vi "doT2.vi"(10 "parameters_recenter":T5={"input_xyz"={"X_um"=0.0, "Y_um"=0.0, "Z_um"=0.0}, "recenter"=FALSE, "recenter_s"=3}, 11 "T1_parameters":T6) -> (0 "triggers":u32[][](array[numeric]), 1 "std_deviation":dbl[](array[numeric]), 2 "T1 curve":cluster{dbl[], "dark_time_us":dbl[]}(graph), 3 "timetags":u32[][](array[numeric]), 5 "position_xyz":T4, 7 "mini_scan":T3)   [LabVIEW 2018]
uses:
  <vilib>/Analysis/NI_AALBase.lvlib
panel:
  in  "parameters_z-scan":T1={"dwell_time_ms"=2.0, "q_steps"=5, "span_um"=1.0, "refocus"=TRUE}
  in  "parameters_xy-scan":T2={"image_size_xy_um"=2.0, "frame_size_xy_px"=7, "dwell_time_ms"=0.5}
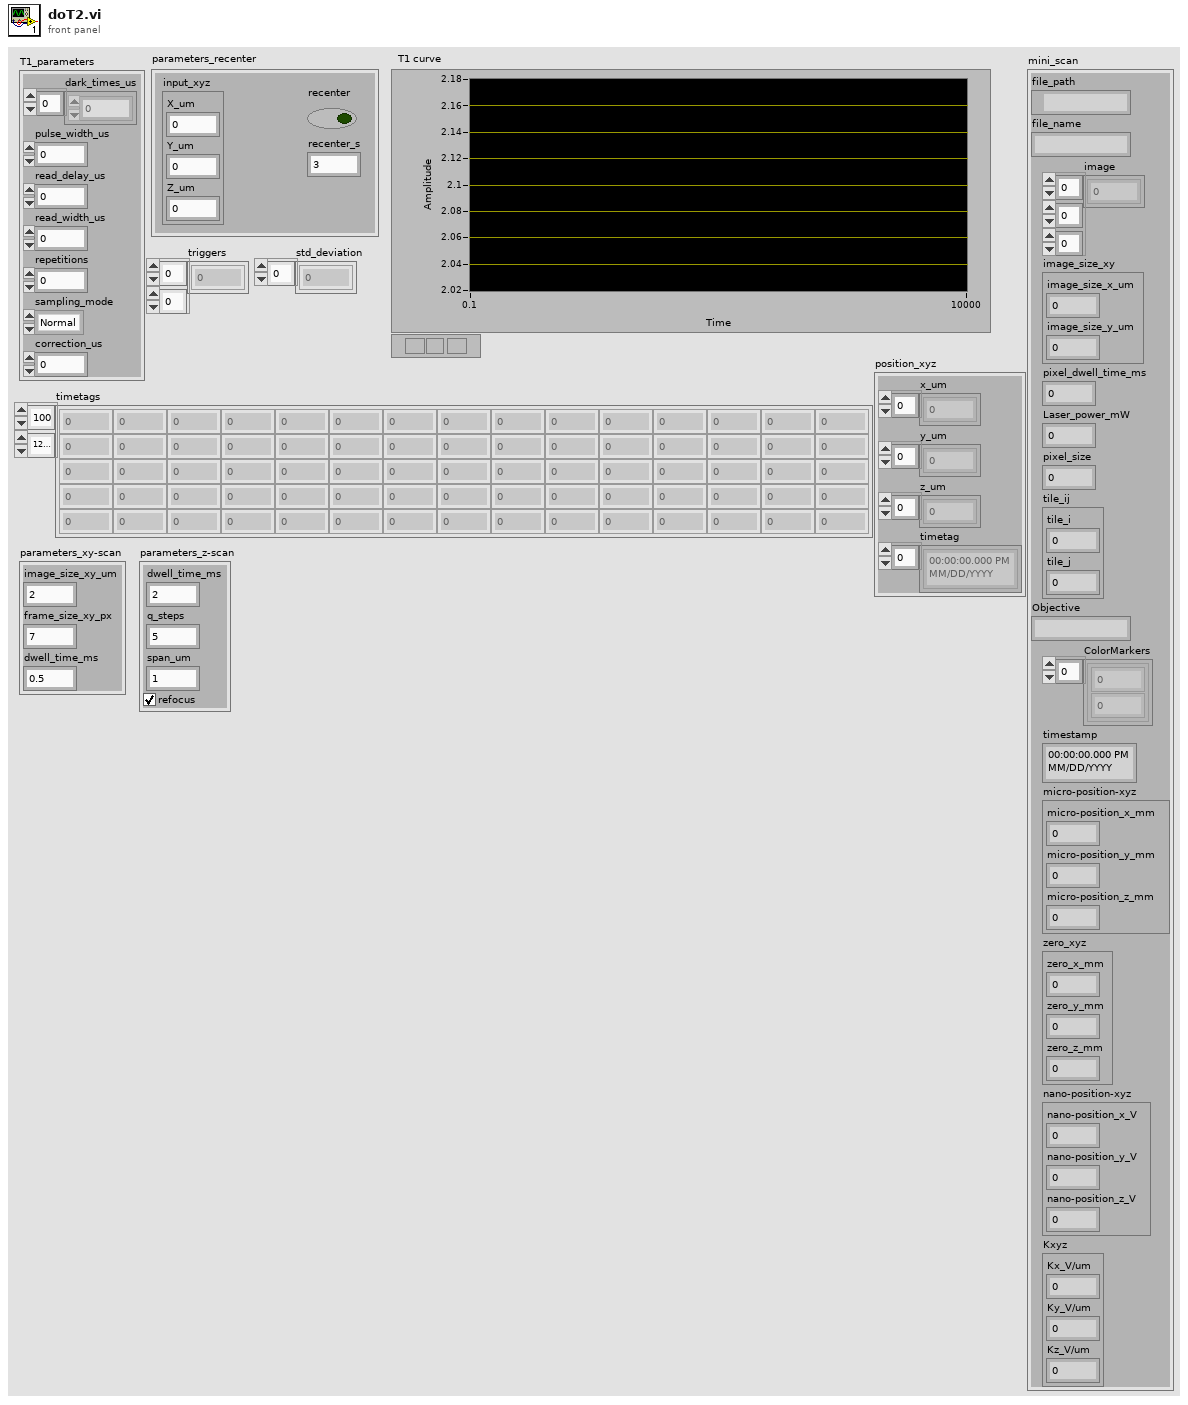
[diagram p1: front panel]
types:
  T1 = cluster{"dwell_time_ms":dbl, "q_steps":u32, "span_um":dbl, "refocus":bool}
  T2 = cluster{"image_size_xy_um":dbl, "frame_size_xy_px":u32, "dwell_time_ms":dbl}
  T3 = cluster{"file_path":path, "file_name":string, "image":dbl[][][], "image_size_xy":cluster{"image_size_x_um":sgl, "image_size_y_um":sgl}, "pixel_dwell_time_ms":sgl, "Laser_power_mW":sgl, "pixel_size":dbl, "tile_ij":cluster{"tile_i":i32, "tile_j":i32}, "Objective":string, "ColorMarkers":cluster{dbl, u32}[], "timestamp":timestamp, "micro-position-xyz":cluster{"micro-position_x_mm":sgl, "micro-position_y_mm":sgl, "micro-position_z_mm":sgl}, "zero_xyz":cluster{"zero_x_mm":dbl, "zero_y_mm":dbl, "zero_z_mm":dbl}, "nano-position-xyz":cluster{"nano-position_x_V":sgl, "nano-position_y_V":sgl, "nano-position_z_V":sgl}, "Kxyz":cluster{"Kx_V/um":sgl, "Ky_V/um":sgl, "Kz_V/um":sgl}}
  T4 = cluster{"x_um":sgl[], "y_um":sgl[], "z_um":sgl[], "timetag":timestamp[]}
  T5 = cluster{"input_xyz":cluster{"X_um":sgl, "Y_um":sgl, "Z_um":sgl}, "recenter":bool, "recenter_s":u32}
  T6 = cluster{"dark_times_us":dbl[], "pulse_width_us":dbl, "read_delay_us":dbl, "read_width_us":dbl, "repetitions":i32, "sampling_mode":enum16{"Normal", "Sweep"}, "correction_us":dbl}
  T7 = cluster{"Instruct Data":i32, "Op Code":i32, "Flags":bool[], "Comments":string, "Time":dbl}[][]
  T8 = cluster{"nano-position_X_um":sgl, "nano-position_Y_um":sgl, "nano-position Z_um":sgl}
  T9 = cluster{"nano-position_X_um":sgl, "nano-position_Y_um":sgl, "nano-position Z_um":sgl}[]
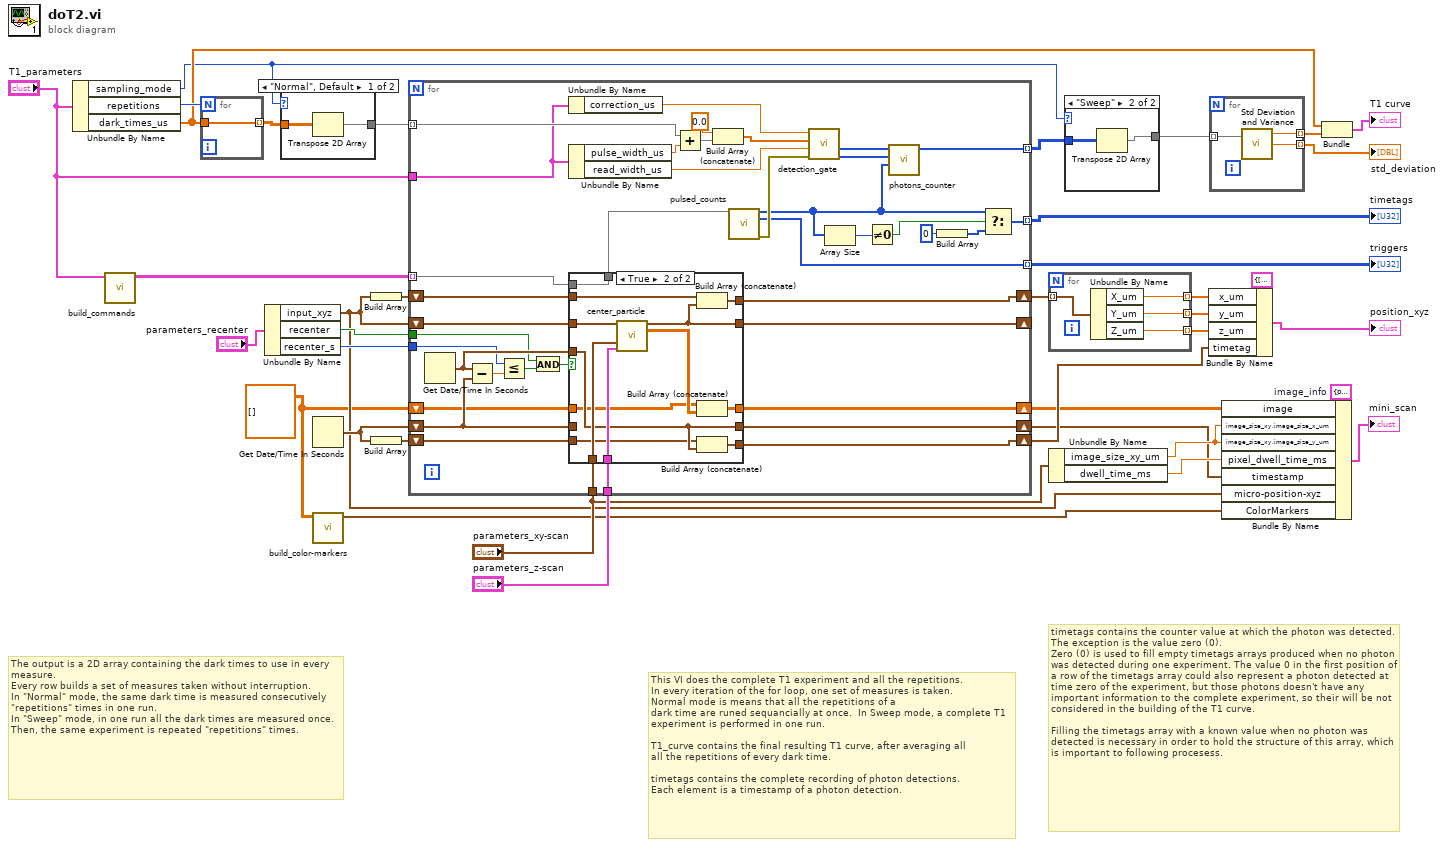
[diagram p0: block diagram]
diagram:
  w2 = dbl[][][] []
  w10 = T3 {"file_path"=path "", "file_name"="", "image"=[], "image_size_xy"={"image_size_x_um"=1.0, "image_size_y_um"=1.0}, "pixel_dwell_time_ms"=1.0, "Laser_power_mW"=1.0, "pixel_size"=0.0, "tile_ij"={"tile_i"=0, "tile_j"=0}, "Objective"="", "ColorMarkers"=[], "timestamp"=timestamp(0 s since 1904-01-01), "micro-position-xyz"={"micro-position_x_mm"=1.0, "micro-position_y_mm"=1.0, "micro-position_z_mm"=1.0}, "zero_xyz"={"zero_x_mm"=0.0, "zero_y_mm"=0.0, "zero_z_mm"=0.0}, "nano-position-xyz"={"nano-position_x_V"=1.0, "nano-position_y_V"=1.0, "nano-position_z_V"=1.0}, "Kxyz"={"Kx_V/um"=1.0, "Ky_V/um"=1.0, "Kz_V/um"=1.0}}  # image_info
  # "timetags contains the counter value at which the photon was detected. The exception is the value zero (0).\nZero (0) is used to fill empty timetags arrays produced when no photon was detected during one experiment. The value 0 in the first position of a row of the timetags array could also represent a photon detected at time zero of the experiment, but those photons doesn't have any important information to the complete experiment, so their will be not considered in the building of the T1 curve.\n\nFilling the timetags array with a known value when no photon was detected is necessary in order to hold the structure of this array, which is important to following procesess."
  # "This VI does the complete T1 experiment and all the repetitions.\nIn every iteration of the for loop, one set of measures is taken.\nNormal mode is means that all the repetitions of a\ndark time are runed sequancially at once.  In Sweep mode, a complete T1 experiment is performed in one run.\n\nT1_curve contains the final resulting T1 curve, after averaging all\nall the repetitions of every dark time.\n\ntimetags contains the complete recording of photon detections.\nEach element is a timestamp of a photon detection."
  # "The output is a 2D array containing the dark times to use in every measure.\nEvery row builds a set of measures taken without interruption.\nIn \"Normal\" mode, the same dark time is measured consecutively \"repetitions\" times in one run.\nIn \"Sweep\" mode, in one run all the dark times are measured once. Then, the same experiment is repeated \"repetitions\" times."
  n1 = Unbundle By Name("T1_parameters") -> ("sampling_mode"=w30:enum16{"Normal", "Sweep"}, "repetitions"=w36:i32, "dark_times_us"=w32:dbl[])
  n2 = call "build_commands.vi"("T1_parameters"="T1_parameters") -> ("instructions_array"=w38:T7)  [unwired: 10 in]
  n3 = for {
    N: w36 -> [_]
    tunnel: w32 -> [w39]
    tunnel: [w39] -> w35 mode=indexing
  }
  n4 = Unbundle By Name("parameters_recenter") -> ("input_xyz"=w3:cluster{"X_um":sgl, "Y_um":sgl, "Z_um":sgl}, "recenter"=w22:bool, "recenter_s"=w23:u32)
  n5 = case shown="\"Normal\", Default" w30 {
    tunnel: w35 -> [w41 w42]
    tunnel: [w40 w42] -> w37
    frame "Normal", Default {
      n6 = Transpose 2D Array(2D array=w41) -> (transposed array=w40:dbl[][])
    }
    frame "Sweep" {
    }
  }
  n7 = Get Date/Time In Seconds() -> (seconds since 1Jan1904=w18:timestamp)
  n8 = call "build_color-markers.vi"("images"=w2) -> ("color_markers"=w1:cluster{dbl, u32}[])  [unwired: 10 in]
  n9 = Build Array(w3) -> (w20:cluster{"X_um":sgl, "Y_um":sgl, "Z_um":sgl}[])
  n10 = Build Array(w18) -> (w19:timestamp[])
  n11 = for {
    tunnel: w38 -> [w62] mode=indexing
    tunnel: w37 -> [w75] mode=indexing
    tunnel: "T1_parameters" -> [w64]
    tunnel: [w76] -> w27 mode=indexing
    tunnel: [w69] -> w26 mode=indexing
    tunnel: [w65] -> w25 mode=indexing
    shift-right: [w60] -> w4
    shift-left: w18 -> [w59]
    tunnel: w23 -> [w56]
    tunnel: w22 -> [w53]
    shift-right: [w49] -> _
    shift-left: w3 -> [w57]
    tunnel: "parameters_xy-scan" -> [w51]
    tunnel: "parameters_z-scan" -> [w50]
    shift-right: [w48] -> w17
    shift-left: w20 -> [w47]
    shift-right: [w46] -> w12
    shift-left: w19 -> [w45]
    shift-right: [w44] -> w9
    shift-left: w2 -> [w43]
    n12 = Get Date/Time In Seconds() -> (seconds since 1Jan1904=w58:timestamp)
    n13 = Subtract(x=w58, y=w59) -> (x-y=w61:dbl)
    n14 = Less Or Equal?(x=w56, y=w61) -> (x <= y?=w55:bool)
    n15 = And(x=w53, y=w55) -> (x .and. y?=w54:bool)
    n16 = Unbundle By Name(w64) -> ("correction_us"=w63:dbl)
    n17 = Unbundle By Name(w64) -> ("pulse_width_us"=w80:dbl, "read_width_us"=w81:dbl)
    n18 = case shown="True" w54 {
      tunnel: w62 -> [w87 w100]
      tunnel: [w87 w100] -> w52
      tunnel: [w83 w93] -> w60
      tunnel: w59 -> [w83 _]
      tunnel: w58 -> [_ w93]
      tunnel: w57 -> [w86 w99]
      tunnel: [w86 w96] -> w49
      tunnel: w51 -> [_ w98]
      tunnel: w50 -> [_ w97]
      tunnel: [w85 w95] -> w48
      tunnel: w47 -> [w85 w94]
      tunnel: [w84 w92] -> w46
      tunnel: w45 -> [w84 w91]
      tunnel: [w82 w90] -> w44
      tunnel: w43 -> [w82 w88]
      frame False {
      }
      frame True {
        n19 = call "center_particle.vi"("input_xyz"=w99, "parameters_xy-scan"=w98, "parameters_z-scan"=w97) -> ("output_xyz"=w96:T8, "mini_scan"=w89:dbl[][])  [unwired: 11 in]
        n20 = Build Array (concatenate)(w94, w96) -> (w95:T9)
        n21 = Build Array (concatenate)(w88, w89) -> (w90:dbl[][][])
        n22 = Build Array (concatenate)(w91, w93) -> (w92:timestamp[])
      }
    }
    n23 = Add(x=w75, y=w80) -> (x+y=w74:dbl[])
    n24 = Build Array (concatenate)(0.0 ("pulse_width_us"), w74) -> (w73:dbl[])
    n25 = call "pulsed_counts.vi"("commands"=w52) -> ("timetags"=w70:u32[], "triggers"=w65:u32[], "Error_out"=w79:errorcluster)  [unwired: 12 in]
    n26 = call "detection_gate.vi"("Error_in"=w79, "read_width_us"=w81, "pulse_period_us"=w73, "correction_us"=w63) -> ("start_read"=w77:u32[], "stop_read"=w78:u32[])  [unwired: 6 in]
    n27 = Array Size(array=w70) -> (size(s)=w66:i32)
    n28 = Not Equal To 0?(x=w66) -> (x != 0?=w71:bool)
    n29 = call "photons_counter.vi"("timetags"=w70, "start_read"=w77, "stop_read"=w78) -> ("photons_counts"=w76:i32[])  [unwired: 8 in]
    n30 = Build Array(u32 0) -> (w67:u32[])
    n31 = Select(t=w70, s=w71, f=w67) -> (s? t:f=w69:u32[])
  }
  "timetags" <- w26
  "triggers" <- w25
  n32 = for {
    tunnel: w17 -> [w104] mode=indexing
    tunnel: [w103] -> w15 mode=indexing
    tunnel: [w102] -> w14 mode=indexing
    tunnel: [w101] -> w13 mode=indexing
    n33 = Unbundle By Name(w104) -> ("X_um"=w103:sgl, "Y_um"=w102:sgl, "Z_um"=w101:sgl)
  }
  n34 = Unbundle By Name("parameters_xy-scan") -> ("image_size_xy_um"=w5:dbl, "dwell_time_ms"=w6:dbl)
  n35 = case shown="\"Sweep\"" w30 {
    tunnel: w27 -> [w105 w107]
    tunnel: [w105 w106] -> w33
    frame "Normal", Default {
    }
    frame "Sweep" {
      n36 = Transpose 2D Array(2D array=w107) -> (transposed array=w106:i32[][])
    }
  }
  n37 = Bundle By Name(cluster=T4 {"x_um"=[], "y_um"=[], "z_um"=[], "timetag"=[]} ("position_xyzt"), "x_um"=w15, "y_um"=w14, "z_um"=w13, "timetag"=w12) -> (→"position_xyz":T4)
  n38 = for {
    tunnel: w33 -> [w110] mode=indexing
    tunnel: [w109] -> w31 mode=indexing
    tunnel: [w108] -> w28 mode=indexing
    n39 = call <vilib>:"Std Deviation and Variance.vi"("X"=w110) -> ("mean"=w109:dbl, "standard deviation"=w108:dbl)  [unwired: 1 in, 1 out]
  }
  "std_deviation" <- w28
  n40 = Bundle By Name(cluster=w10, "image"=w9, "image_size_xy.image_size_x_um"=w5, "image_size_xy.image_size_y_um"=w5, "pixel_dwell_time_ms"=w6, "timestamp"=w4, "micro-position-xyz"=w3, "ColorMarkers"=w1) -> (→"mini_scan":T3)
  n41 = Bundle("dark_times_us"=w32, w31) -> (→"T1 curve":cluster{"dark_times_us":dbl[], dbl[]})  [unwired: 1 in]
